vi "AuthorizationUpdated.vi"(8 "ErrorIn":errorcluster, 11 "ObjectIn":refnum<class "BusAuthorizationUpdated.lvclass">) -> (0 "ErrorOut":errorcluster, 3 "ObjectOut":refnum<class "BusAuthorizationUpdated.lvclass">)   [LabVIEW 2021, in "BusAuthorizationUpdated.lvclass"]
uses:
  BusAuthorizationUpdated.lvclass
  BusAuthorizationUpdated.lvclass/BusAuthorizationUpdated.ctl
  .Externals/Interface_TAF_AutorizationUpdated/IAuthorizationUpdated/IAuthorizationUpdated.lvclass
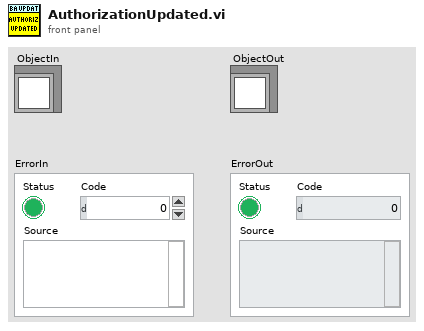
[diagram p1: front panel]
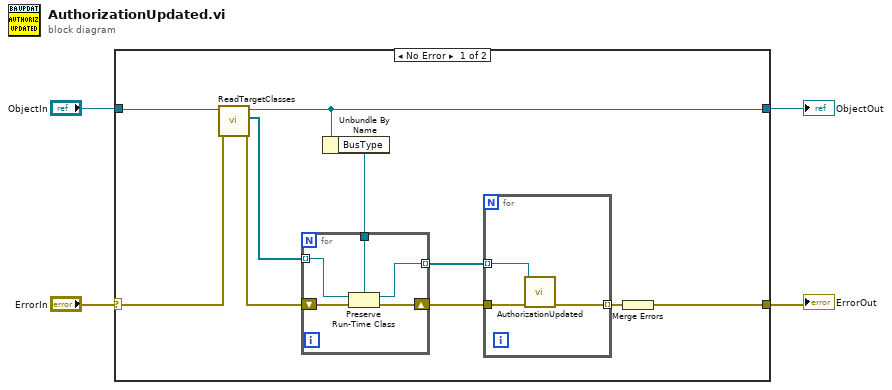
[diagram p0: block diagram]
diagram:
  n1 = case shown="No Error" "ErrorIn" {
    selector: "ErrorIn" -> [w14 w24]
    tunnel: [w11 w24] -> w3
    tunnel: [w9 w23] -> w1
    tunnel: "ObjectIn" -> [w10 w23]
    frame No Error {
      n2 = call-dynamic "ReadTargetClasses.vi"("ErrorIn"=w14, "ReferenceIn"=w10) -> ("ErrorOut"=w13:errorcluster, "TargetClasses"=w7:refnum<class>[], "ReferenceIn"=w9:refnum<class "BusAuthorizationUpdated.lvclass">)  [unwired: 7 in]
      n3 = Unbundle By Name(w9) -> ("BusType"=w8:refnum<class "IAuthorizationUpdated.lvclass">)
      n4 = for {
        tunnel: w7 -> [w17] mode=indexing
        tunnel: [w16] -> w6 mode=indexing
        tunnel: w8 -> [w15]
        shift-right: [w19] -> w12
        shift-left: w13 -> [w18]
        n5 = Preserve Run-Time Class(object in=w17, error in=w18, 2:w15) -> (object out=w16:refnum<class "IAuthorizationUpdated.lvclass">, error out=w19:errorcluster)
      }
      n6 = for {
        tunnel: w6 -> [w20] mode=indexing
        tunnel: w12 -> [w22]
        tunnel: [w21] -> w5 mode=indexing
        n7 = call-dynamic "AuthorizationUpdated.vi"("ErrorIn"=w22, "ObjectIn"=w20) -> ("ErrorOut"=w21:errorcluster)  [unwired: 8 in, 1 out]
      }
      n8 = Merge Errors(w5) -> (w11:errorcluster)
    }
    frame Error {
    }
  }
  "ErrorOut" <- w3
  "ObjectOut" <- w1
